vi "UseEventHandling.vi"() -> ()   [LabVIEW 2009]
uses:
  Instance           3 24Saved   UseEventHandling .vi
  C:/Samples/LabVIEW/UseEventHandling/LabVIEW 2009/UsbDllWrap.dll
panel:
  in  "Stop Events Button":bool
  out "error out":errorcluster
  out "Output:":string
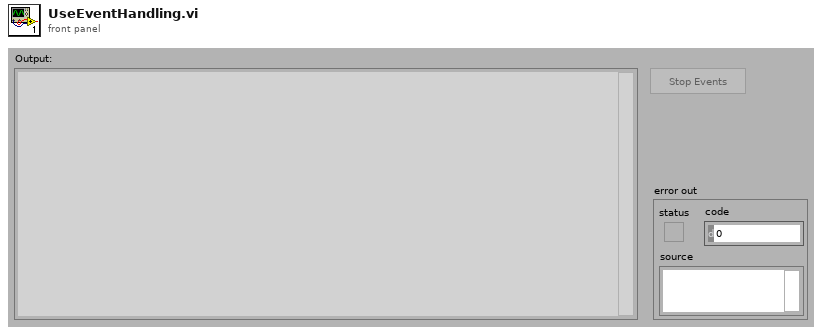
[diagram p1: front panel]
types:
  T1 = enum8{"Enabled", "Disabled", "Disabled and Grayed Out"}
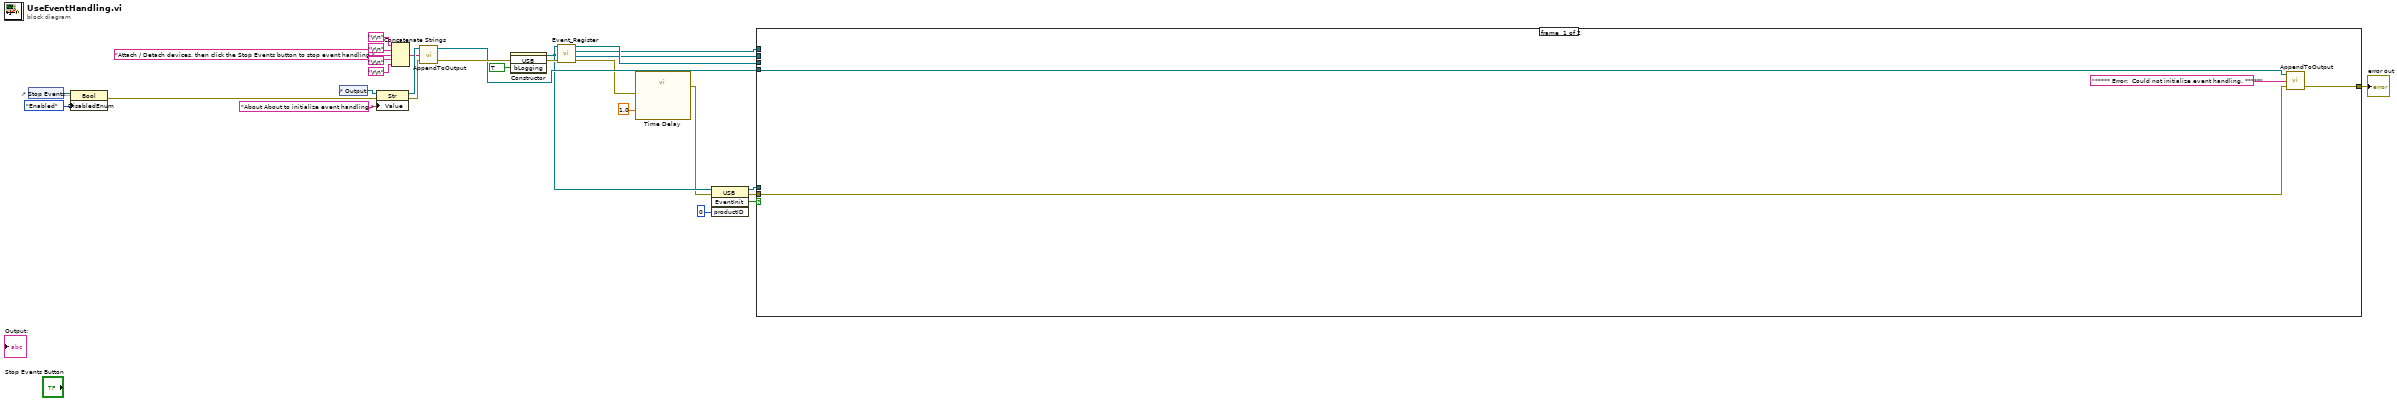
[diagram p0: block diagram]
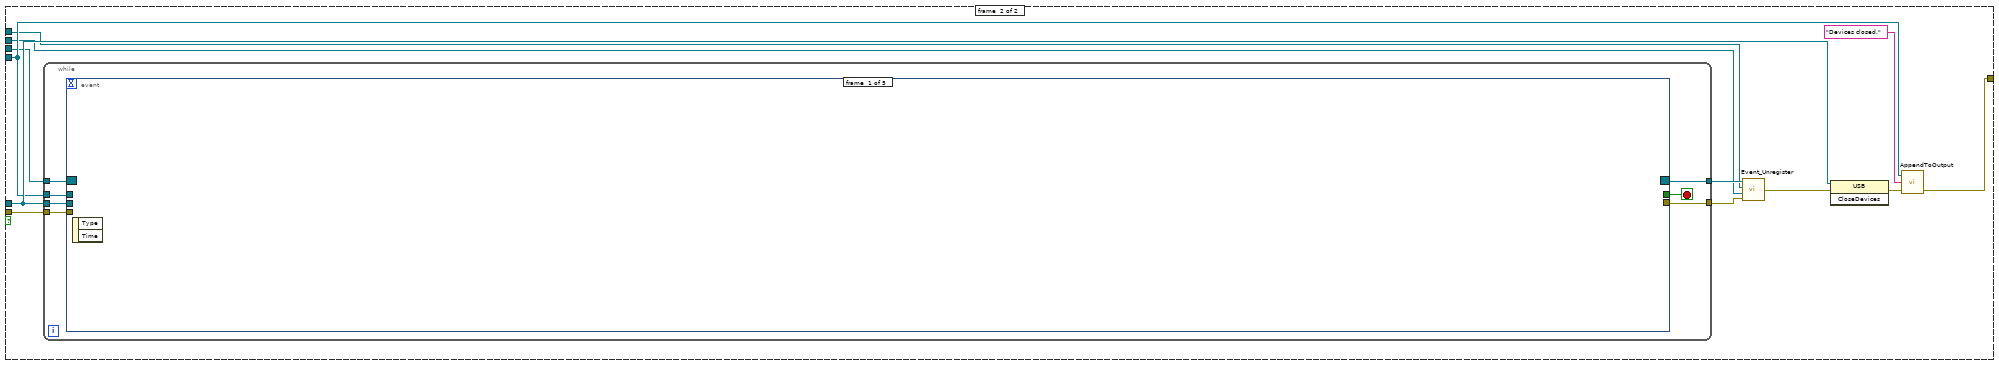
[diagram p2: hidden frame]
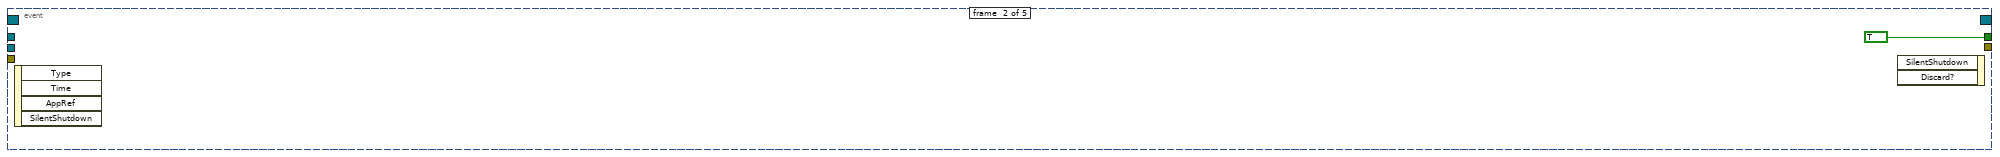
[diagram p3: hidden frame]
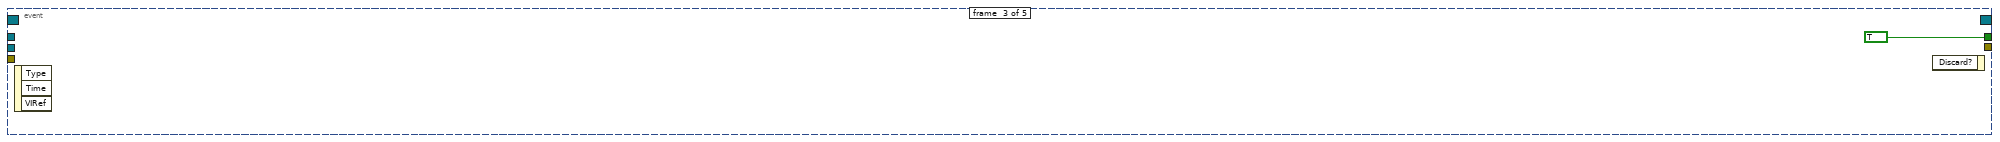
[diagram p4: hidden frame]
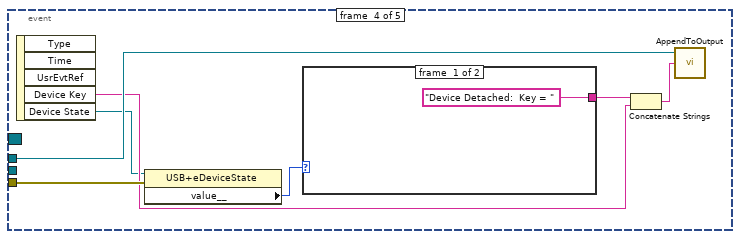
[diagram p5: hidden frame]
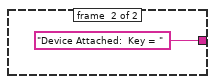
[diagram p6: hidden frame]
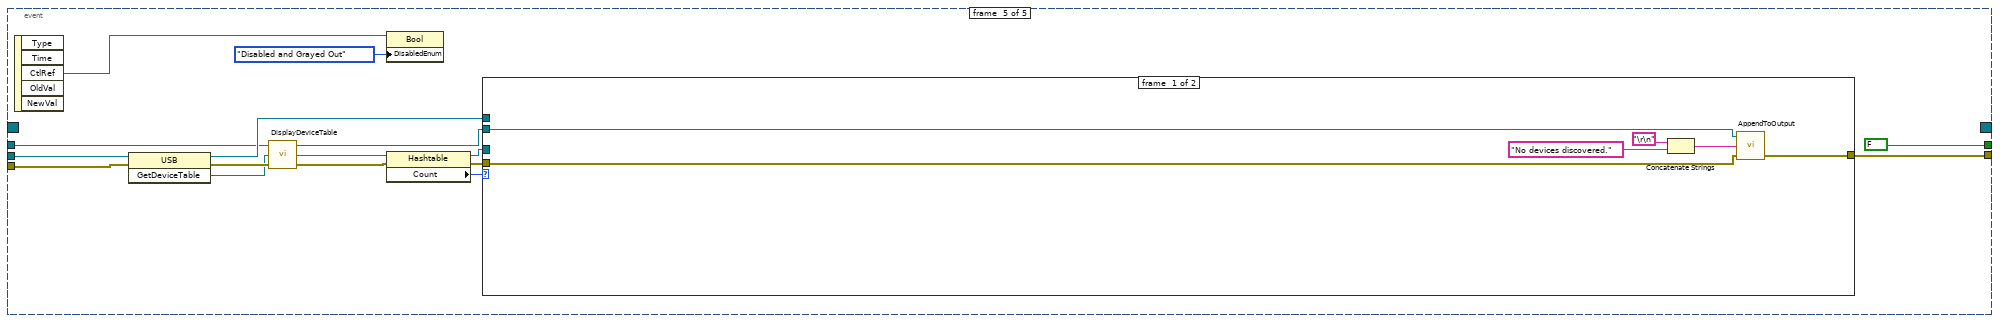
[diagram p7: hidden frame]
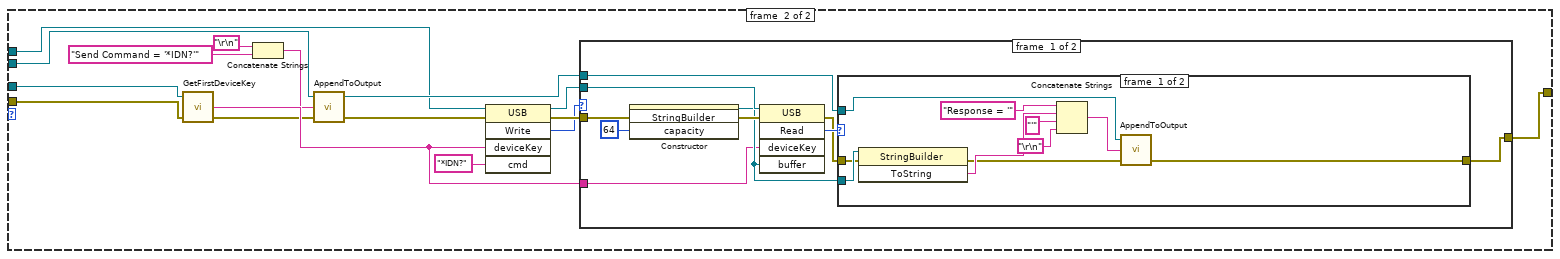
[diagram p8: hidden frame]
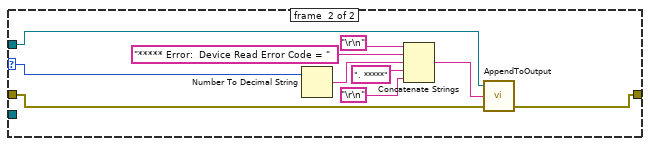
[diagram p9: hidden frame]
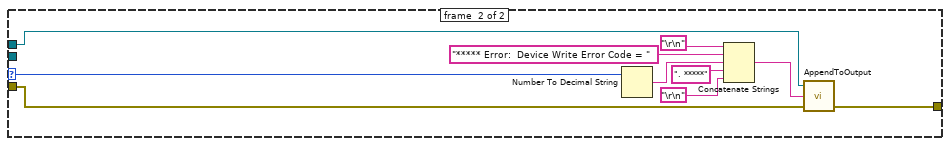
[diagram p10: hidden frame]
diagram:
  n1 = control-ref of="Stop Events Button"() -> (w11:refnum<vi>)
  n2 = property class="Bool"(reference=w11, "DisabledEnum"=T1."Enabled" ("Disabled")) -> (error out=w9:errorcluster)  [unwired: 1 in, 1 out]
  n3 = control-ref of="Output:"() -> (w29:refnum<vi>)
  n4 = property class="Str"(reference=w29, error in=w9, "Value"="About About to initialize event handling.") -> (reference out=w28:refnum<vi>, error out=w25:errorcluster)
  n5 = Concatenate Strings("\r\n", "\r\n", "Attach / Detach devices, then click the Stop Events button to stop event handling." ("Input String"), "\r\n", "\r\n") -> (w18:string)
  n6 = call "AppendToOutput.vi"("error in"=w25, "Input String"=w18, "Output Refnum In"=w28) -> ("error out"=w26:errorcluster, "Output Refnum Out"=w14:refnum<vi>)  [unwired: 1 in]
  n7 = constructor class="USB"(error in=w26, "bLogging"=TRUE) -> (reference out=w7:refnum<k24>, error out=w8:errorcluster)  [unwired: 2 in, 2 out]
  n8 = call "Event_Register.vi"("error in (no error)"=w8, "UsbDllWrap"=w7) -> ("error out"=w3:errorcluster, "Event Callback Refnum"=w4:refnum<k27>, "DeviceStateChangedEvent"=w5:refnum<user-event>, "Event Registration Refnum"=w6:refnum<event-registration>)  [unwired: 2 in]
  n9 = call "Time Delay"("error in (no error)"=w3, "Delay Time (s)"=1.0) -> ("error out"=w2:errorcluster)  [unwired: 9 in]
  n10 = invoke class="USB" method="EventInit"(reference=w7, error in=w2, "productID"=0) -> (reference out=w15:refnum<k24>, error out=w16:errorcluster, "EventInit"=w12:bool)  [unwired: 1 in, 1 out]
  n11 = case shown="True" w12 {
    tunnel: w16 -> [w32 w34]
    tunnel: w15 -> [_ w40]
    tunnel: w14 -> [w31 w38]
    tunnel: [w30 w42] -> w13
    tunnel: w6 -> [_ w37]
    tunnel: w5 -> [_ w36]
    tunnel: w4 -> [_ w35]
    frame #0 {
      n12 = call "AppendToOutput.vi"("error in"=w32, "Input String"="***** Error:  Could not initialize event handling. *****", "Output Refnum In"=w31) -> ("error out"=w30:errorcluster)  [unwired: 1 in, 1 out]
    }
    frame #1 {
      n13 = while {
        tunnel: w38 -> [w51]
        tunnel: w37 -> [w47]
        tunnel: [w46] -> w45
        tunnel: w40 -> [w50]
        tunnel: w34 -> [w49]
        tunnel: [w48] -> w39
        stop <- w52 stop-if-true
        n14 = event shown="[4] \"Stop Events Button\": Value Change" {
          selector: w47 -> [_ _ _ _ _]
          dyn-events: [_ _ _ _ _] -> w46
          timeout: _ -> [_ _ _ _ _]
          tunnel: [_ TRUE TRUE _ FALSE] -> w52
          tunnel: w51 -> [_ _ _ w57 w69]
          tunnel: w50 -> [_ _ _ _ w72]
          tunnel: w49 -> [_ _ _ w58 w71]
          tunnel: [_ _ _ _ w70] -> w48
          event #0 {
            n15 = event-data() -> ()  [unwired: 1 in, 2 out]
          }
          event #1 {
            n16 = event-data() -> ()  [unwired: 1 in, 4 out]
            n17 = event-data() -> ()  [unwired: 3 in, 1 out]
          }
          event #2 {
            n18 = event-data() -> ()  [unwired: 1 in, 3 out]
            n19 = event-data() -> ()  [unwired: 2 in, 1 out]
          }
          event #3 {
            n20 = event-data() -> ("Device Key"=w56:string, "Device State"=w55:refnum<k24>)  [unwired: 1 in, 3 out]
            n21 = property class="USB+eDeviceState"(reference=w55, error in=w58) -> ("value__"=w59:i32)  [unwired: 2 out]
            n22 = case shown="1" w59 {
              tunnel: ["Device Detached:  Key = " "Device Attached:  Key = " ("string")] -> w60
              frame #0 {
              }
              frame #1 {
              }
            }
            n23 = Concatenate Strings(w60, w56) -> (w61:string)
            n24 = call "AppendToOutput.vi"("Input String"=w61, "Output Refnum In"=w57) -> ()  [unwired: 2 in, 2 out]
          }
          event #4 {
            n25 = event-data() -> ("CtlRef"=w78:refnum<vi>)  [unwired: 1 in, 4 out]
            n26 = invoke class="USB" method="GetDeviceTable"(reference=w72, error in=w71) -> (reference out=w73:refnum<k24>, error out=w75:errorcluster, "GetDeviceTable"=w74:refnum<k24>)  [unwired: 1 in]
            n27 = call "DisplayDeviceTable.vi"("error in (no error)"=w75, "Device Table In"=w74, "Output Refnum In"=w69) -> ("error out"=w67:errorcluster, "Device Table Out"=w65:refnum<k24>, "Output Refnum Out"=w76:refnum<vi>)
            n28 = property class="Bool"(reference=w78, "DisabledEnum"=T1."Disabled and Grayed Out" ("Disabled")) -> ()  [unwired: 1 in, 2 out]
            n29 = property class="Hashtable"(reference=w65, error in=w67) -> (reference out=w64:refnum<k24>, error out=w66:errorcluster, "Count"=w68:i32)
            n30 = case shown="1, Default" w68 {
              tunnel: w64 -> [_ w101]
              tunnel: w76 -> [w80 w100]
              tunnel: w66 -> [w82 w99]
              tunnel: w73 -> [_ w91]
              tunnel: [w81 w86] -> w70
              frame #0 {
                n31 = Concatenate Strings("\r\n", "No devices discovered." ("string")) -> (w83:string)
                n32 = call "AppendToOutput.vi"("error in"=w82, "Input String"=w83, "Output Refnum In"=w80) -> ("error out"=w81:errorcluster)  [unwired: 1 in, 1 out]
              }
              frame #1 {
                n33 = call "GetFirstDeviceKey.vi"("error in (no error)"=w99, "Device Table In"=w101) -> ("error out"=w93:errorcluster, "Device Key"=w98:string)  [unwired: 1 in, 1 out]
                n34 = Concatenate Strings("\r\n", "Send Command = '*IDN?'") -> (w89:string)
                n35 = call "AppendToOutput.vi"("error in"=w93, "Input String"=w89, "Output Refnum In"=w100) -> ("error out"=w92:errorcluster, "Output Refnum Out"=w97:refnum<vi>)  [unwired: 1 in]
                n36 = invoke class="USB" method="Write"(reference=w91, error in=w92, "deviceKey"=w98, "cmd"="*IDN?") -> (reference out=w95:refnum<k24>, error out=w96:errorcluster, "Write"=w94:i32)  [unwired: 1 in, 2 out]
                n37 = case shown="0" w94 {
                  selector: w94 -> [_ w136]
                  tunnel: w95 -> [w111 _]
                  tunnel: w96 -> [w108 w134]
                  tunnel: [w104 w133] -> w86
                  tunnel: w97 -> [w103 w132]
                  tunnel: w98 -> [w102 _]
                  frame #0 {
                    n38 = constructor class="StringBuilder"(error in=w108, "capacity"=64) -> (reference out=w106:refnum<k24>, error out=w109:errorcluster)  [unwired: 2 in, 2 out]
                    n39 = invoke class="USB" method="Read"(reference=w111, error in=w109, "deviceKey"=w102, "buffer"=w106) -> (error out=w105:errorcluster, "Read"=w107:i32)  [unwired: 1 in, 3 out]
                    n40 = case shown="0" w107 {
                      selector: w107 -> [_ w126]
                      tunnel: w106 -> [w121 _]
                      tunnel: w105 -> [w120 w123]
                      tunnel: [w113 w122] -> w104
                      tunnel: w103 -> [w112 w124]
                      frame #0 {
                        n41 = invoke class="StringBuilder" method="ToString"(reference=w121, error in=w120) -> (error out=w114:errorcluster, "ToString"=w117:string)  [unwired: 1 in, 1 out]
                        n42 = Concatenate Strings("Response = '", w117, "'", "\r\n") -> (w115:string)
                        n43 = call "AppendToOutput.vi"("error in"=w114, "Input String"=w115, "Output Refnum In"=w112) -> ("error out"=w113:errorcluster)  [unwired: 1 in, 1 out]
                      }
                      frame #1 {
                        n44 = Number To Decimal String(number=w126) -> (decimal integer string=w131:string)  [unwired: 1 in]
                        n45 = Concatenate Strings("\r\n", "***** Error:  Device Read Error Code = ", w131, ". *****", "\r\n") -> (w125:string)
                        n46 = call "AppendToOutput.vi"("error in"=w123, "Input String"=w125, "Output Refnum In"=w124) -> ("error out"=w122:errorcluster)  [unwired: 1 in, 1 out]
                      }
                    }
                  }
                  frame #1 {
                    n47 = Number To Decimal String(number=w136) -> (decimal integer string=w137:string)  [unwired: 1 in]
                    n48 = Concatenate Strings("\r\n", "***** Error:  Device Write Error Code = ", w137, ". *****", "\r\n") -> (w135:string)
                    n49 = call "AppendToOutput.vi"("error in"=w134, "Input String"=w135, "Output Refnum In"=w132) -> ("error out"=w133:errorcluster)  [unwired: 1 in, 1 out]
                  }
                }
              }
            }
          }
        }
      }
      n50 = call "Event_Unregister.vi"("error in"=w39, "Event Callback"=w35, "DeviceStateChangedEvent"=w36, "Event Registration Refnum"=w45) -> ("error out"=w41:errorcluster)
      n51 = invoke class="USB" method="CloseDevices"(reference=w40, error in=w41) -> (error out=w43:errorcluster)  [unwired: 1 in, 2 out]
      n52 = call "AppendToOutput.vi"("error in"=w43, "Input String"="Devices closed." ("string"), "Output Refnum In"=w38) -> ("error out"=w42:errorcluster)  [unwired: 1 in, 1 out]
    }
  }
  "error out" <- w13
